vi "Get Mantissa and Exponent (SGL).vi"(11 "Input":fxp<+,32,32>) -> (1 "sign":bool, 2 "Exponent":fxp<+/-,8,8>, 3 "FXP Part":fxp<+/-,25,2> format="%.25g")   [LabVIEW 2012]
doc: "Note: This VI extracts exponent and mantissa of <b> positive </b> integer."
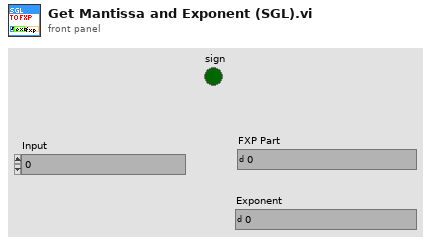
[diagram p1: front panel]
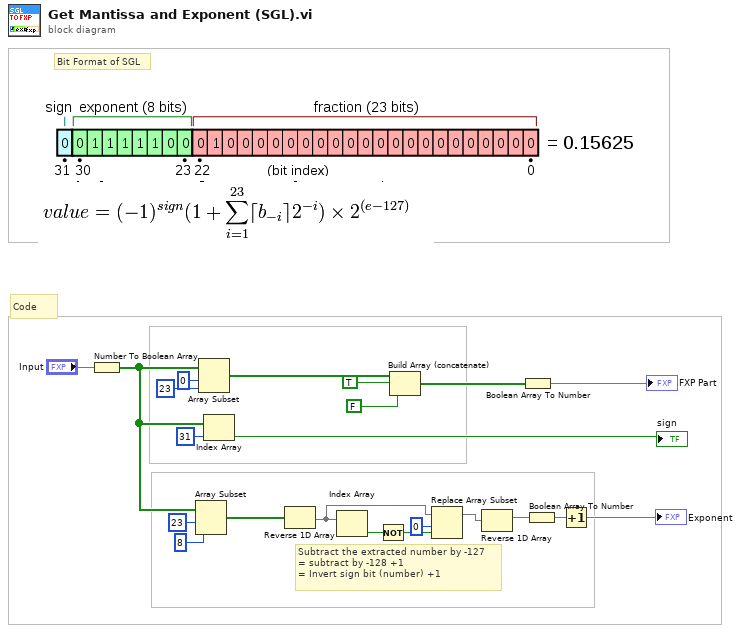
[diagram p0: block diagram]
diagram:
  # "Code"
  # "Bit Format of SGL"
  # "Subtract the extracted number by -127\n= subtract by -128 +1\n= Invert sign bit (number) +1"
  n1 = Number To Boolean Array(number="Input") -> (Boolean array=w14:bool[])
  n2 = Array Subset(array=w14, index=23, length=8) -> (w12:bool[])
  n3 = Array Subset(array=w14, index=0, length=23) -> (w18:bool[])
  n4 = Index Array(array=w14, index=31) -> (element=→"sign":bool)
  n5 = Reverse 1D Array(array=w12) -> (reversed array=w8:bool[])
  n6 = Index Array(array=w8) -> (element=w11:bool)  [unwired: 1 in]
  n7 = Not(x=w11) -> (.not. x?=w10:bool)
  n8 = Build Array (concatenate)(w18, TRUE, FALSE ("element")) -> (w17:bool[])
  n9 = Replace Array Subset(array=w8, new element=w10, index=0) -> (w7:bool[])
  n10 = Reverse 1D Array(array=w7) -> (reversed array=w6:bool[])
  n11 = Boolean Array To Number(Boolean array=w17) -> (number=→"FXP Part":fxp<+/-,25,2>)
  n12 = Boolean Array To Number(Boolean array=w6) -> (number=w5:fxp<+/-,8,8>)
  n13 = Increment(x=w5) -> (x+1=→"Exponent":fxp<+/-,8,8>)
